vi "Configure.vi"(8 "error in (no error)":errorcluster, 10 "Device Configurations":T1={"Trace Config"={"Trace Selection"=enum."Trace A", "Roll Avg"=2.0}, "Measurement Config"={"Wavelength"={"Center Wavelength (nm)"=1550.0, "Span (nm)"=10.0}, "Sampling"={"Mode"=enum."Auto", "No. Samples"=5501}, "Sens-Resolution"={"Resolution (nm)"=0.0}, "Main Scale"={"Reference Level (dBm)"=0.0, "Log Scale (dB/Div)"=0.0}}}, 11 "Yokogawa AQ6370D in":refnum<class "Yokogawa AQ6370D.lvclass">) -> (0 "error out":errorcluster, 3 "Yokogawa AQ6370D out":refnum<class "Yokogawa AQ6370D.lvclass">)   [LabVIEW 2018, in "Yokogawa AQ6370D.lvlib" / "Yokogawa AQ6370D.lvclass"]
uses:
  Yokogawa AQ6370D.lvclass
  PPLs/Optical Spectrum Analyzer/Parent/OSA.lvlibp/Custom Controls/cls_Device Configurations.ctl
  PPLs/Optical Spectrum Analyzer/Parent/OSA.lvlibp/Custom Controls/enm_Trace Selection.ctl
  Yokogawa AQ6370D.lvclass/Yokogawa AQ6370D.ctl
  PPLs/Optical Spectrum Analyzer/Parent/OSA.lvlibp/Optical Spectrum Analyzer.lvclass
  C:/Projects/LabVIEW/PPLs/Optical Spectrum Analyzer/Parent/OSA.lvlibp/Optical Spectrum Analyzer.lvclass
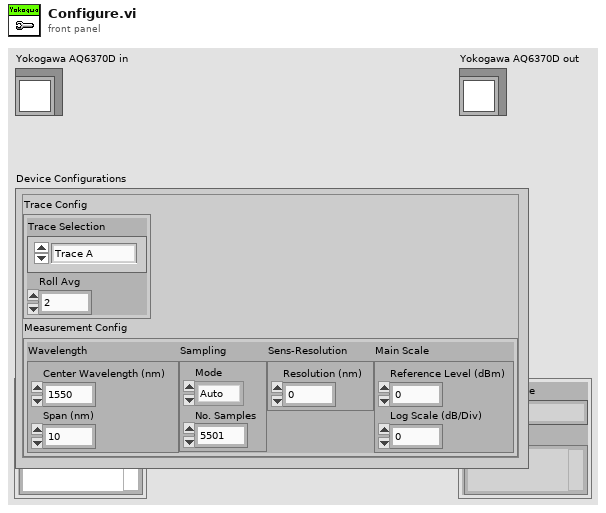
[diagram p1: front panel]
types:
  T1 = typedef "OSA.lvlibp/Optical Spectrum Analyzer.lvclass/cls_Device Configurations.ctl" = cluster{"Trace Config":cluster{"Trace Selection":T2, "Roll Avg":dbl}, "Measurement Config":cluster{"Wavelength":cluster{"Center Wavelength (nm)":dbl, "Span (nm)":dbl}, "Sampling":cluster{"Mode":enum16{"Auto", "Manual"}, "No. Samples":u32}, "Sens-Resolution":cluster{"Resolution (nm)":dbl}, "Main Scale":cluster{"Reference Level (dBm)":dbl, "Log Scale (dB/Div)":dbl}}}
  T2 = typedef "OSA.lvlibp/Optical Spectrum Analyzer.lvclass/enm_Trace Selection.ctl" = enum16{"Trace A", "Trace B", "Trace C", "Trace D", "Trace E", "Trace F", "Trace G"}
  T3 = cluster{"Wavelength":cluster{"Center Wavelength (nm)":dbl, "Span (nm)":dbl}, "Sampling":cluster{"Mode":enum16{"Auto", "Manual"}, "No. Samples":u32}, "Sens-Resolution":cluster{"Resolution (nm)":dbl}, "Main Scale":cluster{"Reference Level (dBm)":dbl, "Log Scale (dB/Div)":dbl}}
  T4 = cluster{"Center Wavelength (nm)":dbl, "Span (nm)":dbl}
  T5 = cluster{"Mode":enum16{"Auto", "Manual"}, "No. Samples":u32}
  T6 = cluster{"Reference Level (dBm)":dbl, "Log Scale (dB/Div)":dbl}
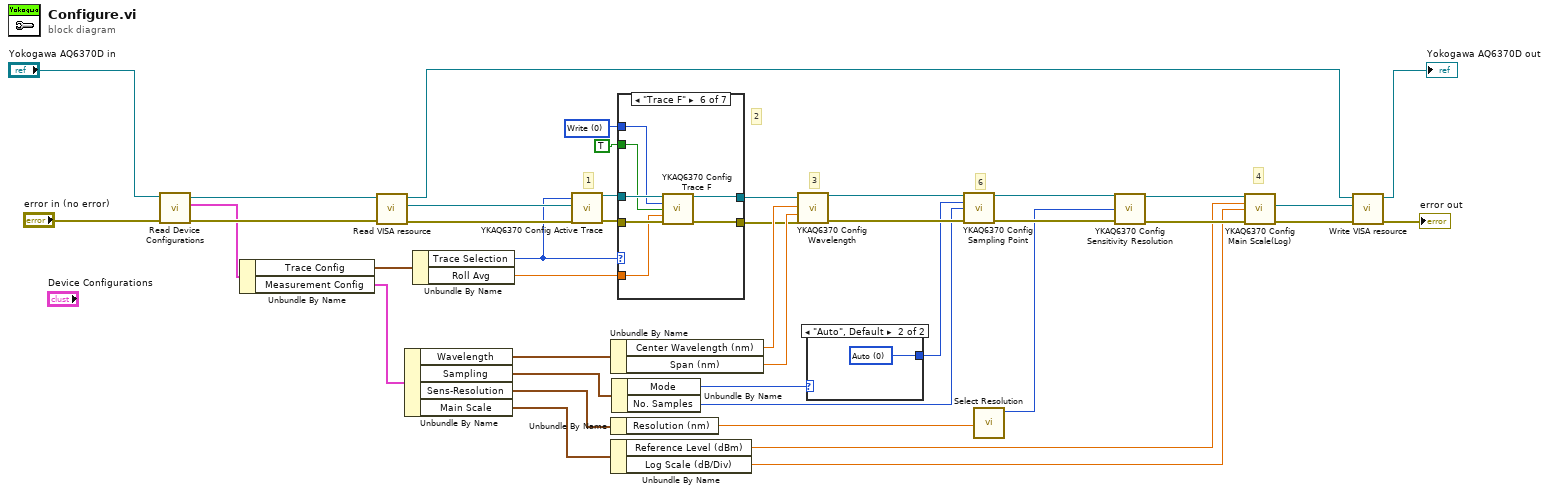
[diagram p0: block diagram]
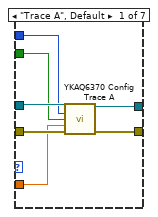
[diagram p2: hidden frame]
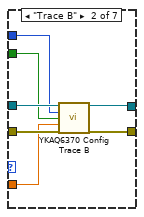
[diagram p3: hidden frame]
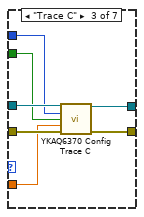
[diagram p4: hidden frame]
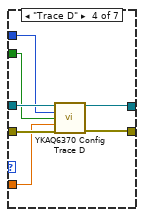
[diagram p5: hidden frame]
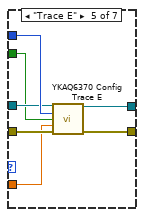
[diagram p6: hidden frame]
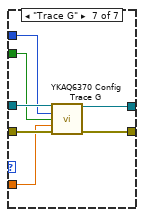
[diagram p7: hidden frame]
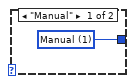
[diagram p8: hidden frame]
diagram:
  w17 = u16 0 items=["Write", "Fix", "Max Hold", "Min Hold", "Roll Average"] ("Trace A ATTR")
  # "6"
  # "4"
  # "3"
  # "2"
  # "1"
  n1 = call "Read Device Configurations.vi"("error in (no error)"="error in (no error)", "Optical Spectrum Analyzer in"="Yokogawa AQ6370D in") -> ("error out"=w2:errorcluster, "Device Configurations"=w1:T1, "Optical Spectrum Analyzer out"=w4:refnum<class "Yokogawa AQ6370D.lvclass">)  [unwired: 7 in]
  n2 = Unbundle By Name(w1) -> ("Trace Config"=w13:cluster{"Trace Selection":T2, "Roll Avg":dbl}, "Measurement Config"=w36:T3)
  n3 = call "Read VISA resource.vi"("error in (no error)"=w2, "Yokogawa AQ6370D in"=w4) -> ("error out"=w41:errorcluster, "VISA resource"=w37:refnum<visa-resource-name>, "Yokogawa AQ6370D out"=w39:refnum<class "Yokogawa AQ6370D.lvclass">)  [unwired: 7 in]
  n4 = Unbundle By Name(w36) -> ("Wavelength"=w35:T4, "Sampling"=w10:T5, "Sens-Resolution"=w9:cluster{"Resolution (nm)":dbl}, "Main Scale"=w8:T6)
  n5 = Unbundle By Name(w13) -> ("Trace Selection"=w12:T2, "Roll Avg"=w11:dbl)
  n6 = call <instrlib>:"YKAQ6370 Config Active Trace.vi"("VISA resource name"=w37, "Active Trace (0: Trace A)"=w12, "error in (no error)"=w41) -> ("VISA resource name out"=w18:refnum<visa-resource-name>, "error out"=w19:errorcluster)  [unwired: 11 in]
  n7 = Unbundle By Name(w35) -> ("Center Wavelength (nm)"=w34:dbl, "Span (nm)"=w33:dbl)
  n8 = Unbundle By Name(w9) -> ("Resolution (nm)"=w7:dbl)
  n9 = Unbundle By Name(w8) -> ("Reference Level (dBm)"=w21:dbl, "Log Scale (dB/Div)"=w20:dbl)
  n10 = Unbundle By Name(w10) -> ("Mode"=w29:enum16{"Auto", "Manual"}, "No. Samples"=w30:u32)
  n11 = case shown="\"Trace F\"" w12 {
    tunnel: w18 -> [w47 w55 w62 w69 w75 w83 w90]
    tunnel: w19 -> [w48 w54 w60 w67 w73 w82 w88]
    tunnel: [w46 w53 w61 w68 w74 w81 w89] -> w15
    tunnel: [w45 w52 w59 w66 w72 w80 w87] -> w14
    tunnel: w17 -> [w44 w51 w58 w65 w76 w79 w86]
    tunnel: TRUE ("Disp / Blank") -> [w43 w50 w57 w64 w71 w78 w85]
    tunnel: w11 -> [w42 w49 w56 w63 w70 w77 w84]
    frame "Trace A", Default {
      n12 = call <instrlib>:"YKAQ6370 Config Trace A.vi"("VISA resource name"=w47, "Trace A ATTR  (0: Write)"=w44, "Disp / Blank (T: Disp)"=w43, "Roll Average (2)"=w42, "error in (no error)"=w48) -> ("VISA resource name out"=w46:refnum<visa-resource-name>, "error out"=w45:errorcluster)  [unwired: 9 in]
    }
    frame "Trace B" {
      n13 = call <instrlib>:"YKAQ6370 Config Trace B.vi"("VISA resource name"=w55, "Trace B ATTR  (0: Write)"=w51, "Disp / Blank (F: Blank)"=w50, "Roll Average (2)"=w49, "error in (no error)"=w54) -> ("VISA resource name out"=w53:refnum<visa-resource-name>, "error out"=w52:errorcluster)  [unwired: 9 in]
    }
    frame "Trace C" {
      n14 = call <instrlib>:"YKAQ6370 Config Trace C.vi"("VISA resource name"=w62, "Trace C ATTR (1: Fix)"=w58, "Disp / Blank (F: Blank)"=w57, "Roll Average (2)"=w56, "error in (no error)"=w60) -> ("VISA resource name out"=w61:refnum<visa-resource-name>, "error out"=w59:errorcluster)  [unwired: 9 in]
    }
    frame "Trace D" {
      n15 = call <instrlib>:"YKAQ6370 Config Trace D.vi"("VISA resource name"=w69, "Trace D ATTR  (0: Write)"=w65, "Disp / Blank (F: Blank)"=w64, "Roll Average (2)"=w63, "error in (no error)"=w67) -> ("VISA resource name out"=w68:refnum<visa-resource-name>, "error out"=w66:errorcluster)  [unwired: 9 in]
    }
    frame "Trace E" {
      n16 = call <instrlib>:"YKAQ6370 Config Trace E.vi"("VISA resource name"=w75, "Trace E ATTR  (0: Write)"=w76, "Disp / Blank (F: Blank)"=w71, "Roll Average (2)"=w70, "error in (no error)"=w73) -> ("VISA resource name out"=w74:refnum<visa-resource-name>, "error out"=w72:errorcluster)  [unwired: 9 in]
    }
    frame "Trace F" {
      n17 = call <instrlib>:"YKAQ6370 Config Trace F.vi"("VISA resource name"=w83, "Trace F ATTR (1: Fix)"=w79, "Disp / Blank (1: Blank)"=w78, "Roll Average (2)"=w77, "error in (no error)"=w82) -> ("VISA resource name out"=w81:refnum<visa-resource-name>, "error out"=w80:errorcluster)  [unwired: 9 in]
    }
    frame "Trace G" {
      n18 = call <instrlib>:"YKAQ6370 Config Trace G.vi"("VISA resource name"=w90, "Trace G ATTR (1: Fix)"=w86, "Disp / Blank (F: Blank)"=w85, "Roll Average (2)"=w84, "error in (no error)"=w88) -> ("VISA resource name out"=w89:refnum<visa-resource-name>, "error out"=w87:errorcluster)  [unwired: 9 in]
    }
  }
  n19 = call <instrlib>:"YKAQ6370 Config Wavelength.vi"("VISA resource name"=w15, "Center/Start (1150.000)"=w34, "Span/Stop  (1100.000)"=w33, "error in (no error)"=w14) -> ("VISA resource name out"=w32:refnum<visa-resource-name>, "error out"=w31:errorcluster)  [unwired: 10 in]
  n20 = case shown="\"Auto\", Default" w29 {
    tunnel: [w91 w92] -> w28
    frame "Manual" {
      w91 = u16 1 items=["Auto", "Manual"] ("Sampling Point (0: Auto)")
    }
    frame "Auto", Default {
      w92 = u16 0 items=["Auto", "Manual"] ("Sampling Point (0: Auto)")
    }
  }
  n21 = call <instrlib>:"YKAQ6370 Config Sampling Point.vi"("VISA resource name"=w32, "Sampling Point (0: Auto)"=w28, "Sampling Point (5501)"=w30, "error in (no error)"=w31) -> ("VISA resource name out"=w27:refnum<visa-resource-name>, "error out"=w26:errorcluster)  [unwired: 10 in]
  n22 = call "Select Resolution.vi"("Resolution (nm)"=w7) -> ("Resolution (6: 1.000nm)"=w6:u16)  [unwired: 9 in, 1 out]
  n23 = call <instrlib>:"YKAQ6370 Config Sensitivity Resolution.vi"("VISA resource name"=w27, "Resolution (6: 1.000nm)"=w6, "error in (no error)"=w26) -> ("VISA resource name out"=w25:refnum<visa-resource-name>, "error out"=w24:errorcluster)  [unwired: 11 in]
  n24 = call <instrlib>:"YKAQ6370 Config Main Scale(Log).vi"("VISA resource name"=w25, "Reference Level (-10.0)"=w21, "Log Scale (10.0)"=w20, "error in (no error)"=w24) -> ("VISA resource name out"=w22:refnum<visa-resource-name>, "error out"=w23:errorcluster)  [unwired: 10 in]
  n25 = call "Write VISA resource.vi"("error in (no error)"=w23, "VISA resource"=w22, "Yokogawa AQ6370D in"=w39) -> ("error out"=→"error out":errorcluster, "Yokogawa AQ6370D out"=→"Yokogawa AQ6370D out":refnum<class "Yokogawa AQ6370D.lvclass">)  [unwired: 7 in]
